vi "Start.vi"(9 "Team In":refnum<class "Team.lvclass">, 11 "Square in":refnum<class "Square.lvclass">) -> (1 "Team":refnum<class "Team.lvclass">, 3 "Square out":refnum<class "Square.lvclass">)   [LabVIEW 2020, in "SquareBattle.lvlib" / "Square.lvclass"]
doc: "This VI is called when the square is being added to the game, either during the initial placement (round 0) or from a replication. This gives an opportunity for the square to register with the team if necessary and have it state initialized."
uses:
  Square.lvclass
  Team/Team.lvclass
  Square.lvclass/Square.ctl
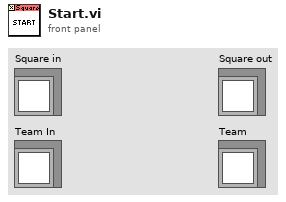
[diagram p1: front panel]
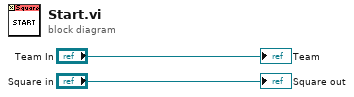
[diagram p0: block diagram]
diagram:
  "Square out" <- "Square in"
  "Team" <- "Team In"
